vi "Unwrap (SubVI).vi"(1 "phase in":dbl[](array[numeric])) -> (8 "phase out":dbl[](array[numeric]))   [LabVIEW 2012]
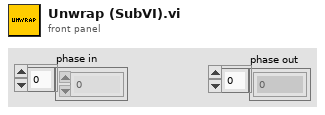
[diagram p1: front panel]
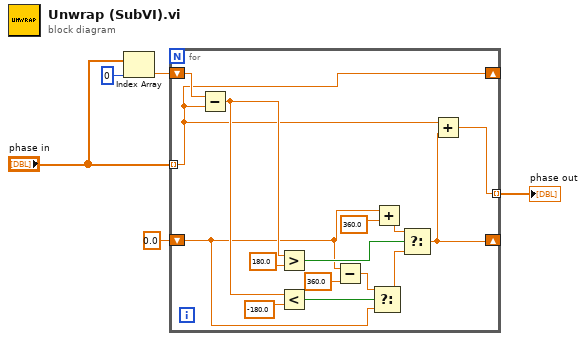
[diagram p0: block diagram]
diagram:
  n1 = Index Array(array="phase in", index=0) -> (element=w2:dbl)
  n2 = for {
    tunnel: "phase in" -> [w8] mode=indexing
    shift-right: [w8] -> _
    shift-left: w2 -> [w20]
    tunnel: [w9] -> w5 mode=indexing
    shift-right: [w7] -> _
    shift-left: 0.0 -> [w6]
    n3 = Subtract(x=w20, y=w8) -> (x-y=w11:dbl)
    n4 = Greater?(x=w11, y=180.0) -> (0:w18:bool)
    n5 = Less?(x=w11, y=-180.0) -> (x < y?=w17:bool)
    n6 = Subtract(x=w6, y=360.0) -> (x-y=w13:dbl)
    n7 = Select(t=w13, s=w17, f=w6) -> (s? t:f=w12:dbl)
    n8 = Add(x=w6, y=360.0) -> (x+y=w15:dbl)
    n9 = Select(t=w15, s=w18, f=w12) -> (s? t:f=w7:dbl)
    n10 = Add(x=w8, y=w7) -> (x+y=w9:dbl)
  }
  "phase out" <- w5
